vi "GV FIFO timeout.vi"() -> ()   [LabVIEW 2017]
panel:
  out "FIFO timeout":i32
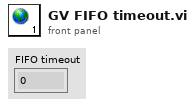
[diagram p1: front panel]
diagram:
